vi "VI Tree.vi"   [LabVIEW 2021, in "VI-Hacker.lvlib"]
uses:
  VI-Hacker.lvlib
  TypeDefs/Block BDPW.ctl
  TypeDefs/Block vers.ctl
  TypeDefs/Block.ctl
  TypeDefs/Content.ctl
  TypeDefs/RSRC_Header.ctl
  TypeDefs/RSRC_Id.ctl
  TypeDefs/RSRC_Info.ctl
types:
  T1 = typedef "VI-Hacker.lvlib/RSRC_Info.ctl" = cluster{"Int1":i32, "Int2":i32, "Int3":i32, "DataOffset":i32, "Int4":i32}
  T2 = typedef "VI-Hacker.lvlib/RSRC_Id.ctl" = cluster{"Name":u32, "Count":u32, "Offset":i32}
  T3 = typedef "VI-Hacker.lvlib/RSRC_Header.ctl" = cluster{"RSRC\\r\\n\\xx\\xx":u64, "LVINLBVW":u64, "RSRCOffset":i32, "RSRCSize":i32, "DataOffset":i32, "DataSize":i32}
  T4 = typedef "VI-Hacker.lvlib/Content.ctl" = cluster{"Binary Data":string, "Blocks":T5[]}
  T5 = typedef "VI-Hacker.lvlib/Block.ctl" = cluster{"Name":string, "Offset":i32, "Size":i32, "LenSize":i32}
  T6 = typedef "VI-Hacker.lvlib/Block vers.ctl" = cluster{"Version":cluster{"Major":u8, "Minor":u8, "Fix":u8, "Build":u8}, "Stage":enum8{"Development", "Alpha", "Beta", "Release"}, "Flags":u16, "VersionString":string, "VersionInfo":string}
  T7 = typedef "VI-Hacker.lvlib/Block BDPW.ctl" = cluster{"Pswrd (md5)":string, "Hash1 (md5)":string, "Hash2 (md5)":string}
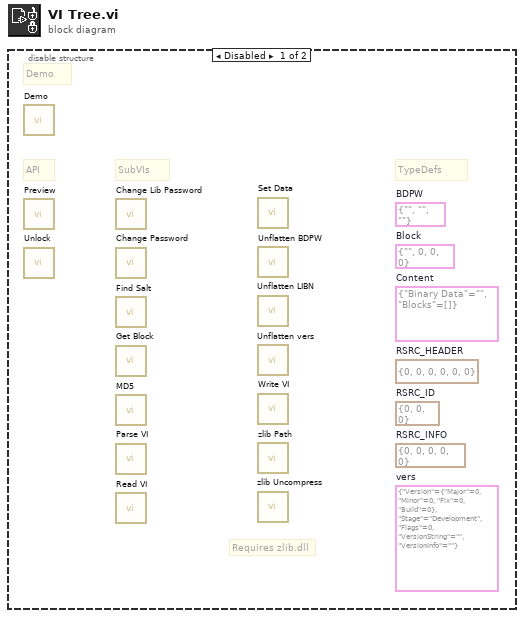
[diagram p0: block diagram]
diagram:
  n1 = disable-structure shown="Disabled" {
    frame Disabled {
      (unwired) T1 {"Int1"=0, "Int2"=0, "Int3"=0, "DataOffset"=0, "Int4"=0}  # RSRC_INFO
      (unwired) T2 {"Name"=0, "Count"=0, "Offset"=0}  # RSRC_ID
      (unwired) T3 {"RSRC\\r\\n\\xx\\xx"=0, "LVINLBVW"=0, "RSRCOffset"=0, "RSRCSize"=0, "DataOffset"=0, "DataSize"=0}  # RSRC_HEADER
      (unwired) T4 {"Binary Data"="", "Blocks"=[]}  # Content
      (unwired) T5 {"Name"="", "Offset"=0, "Size"=0, "LenSize"=0}  # Block
      (unwired) T6 {"Version"={"Major"=0, "Minor"=0, "Fix"=0, "Build"=0}, "Stage"=enum."Development", "Flags"=0, "VersionString"="", "VersionInfo"=""}  # vers
      (unwired) T7 {"Pswrd (md5)"="", "Hash1 (md5)"="", "Hash2 (md5)"=""}  # BDPW
      # "Requires zlib.dll"
      # "Demo"
      # "TypeDefs"
      # "SubVIs"
      # "API"
      n2 = call "Demo.vi"() -> ()  [unwired: 12 in]
      n3 = call "Preview.vi"() -> ()  [unwired: 11 in, 1 out]
      n4 = call "Unlock.vi"() -> ()  [unwired: 10 in, 2 out]
      n5 = call "Change Lib Password.vi"() -> ()  [unwired: 9 in, 3 out]
      n6 = call "Change Password.vi"() -> ()  [unwired: 10 in, 2 out]
      n7 = call "Find Salt.vi"() -> ()  [unwired: 8 in, 4 out]
      n8 = call "Get Block.vi"() -> ()  [unwired: 7 in, 5 out]
      n9 = call "MD5.vi"() -> ()  [unwired: 10 in, 2 out]
      n10 = call "Parse VI.vi"() -> ()  [unwired: 10 in, 2 out]
      n11 = call "Read VI.vi"() -> ()  [unwired: 10 in, 2 out]
      n12 = call "Set Data.vi"() -> ()  [unwired: 10 in, 2 out]
      n13 = call "Unflatten BDPW.vi"() -> ()  [unwired: 10 in, 2 out]
      n14 = call "Unflatten LIBN.vi"() -> ()  [unwired: 9 in, 3 out]
      n15 = call "Unflatten vers.vi"() -> ()  [unwired: 10 in, 2 out]
      n16 = call "Write VI.vi"() -> ()  [unwired: 10 in, 2 out]
      n17 = call "zlib Path.vi"() -> ()  [unwired: 9 in, 3 out]
      n18 = call "zlib Uncompress.vi"() -> ()  [unwired: 9 in, 3 out]
    }
    frame Enabled {
    }
  }
